vi "SM_DI-DAQInstrument.vi"(7 "DI TaskName":string, 8 "error in (no error)":errorcluster, 11 "DAQ Process AppData":T1) -> (0 "error out":errorcluster)   [LabVIEW 2017, in "DAQ.lvclass"]
doc: "Developed by Kevin Thompson\nkevin@thompsonengineering.net\n\nCopyright 2018-2020\nThompson Engineering, LLC"
uses:
  DAQ.lvclass
  Process_DAQ SM AppData--cluster.ctl
  DataTypes/TD DAQ Settings--cluster.ctl
  DataTypes/TD DI Instrument Settings--cluster.ctl
  DataTypes/TD AI Instrument Settings--cluster.ctl
  DataTypes/TD AI InstSettings--cluster.ctl
  TD SimAI Ranges--cluster.ctl
  <vilib>/TELLC/Dynamic CVT API/TD Dynamic CVT DVR--ref.ctl
  TD local raw DI Data--cluster.ctl
  <vilib>/DAQmx/read.llb/DAQmx Read (Digital 1D Bool NChan 1Samp 1Line).vi
  <vilib>/DAQmx/miscellaneous.llb/DAQmx Fill In Error Info.vi
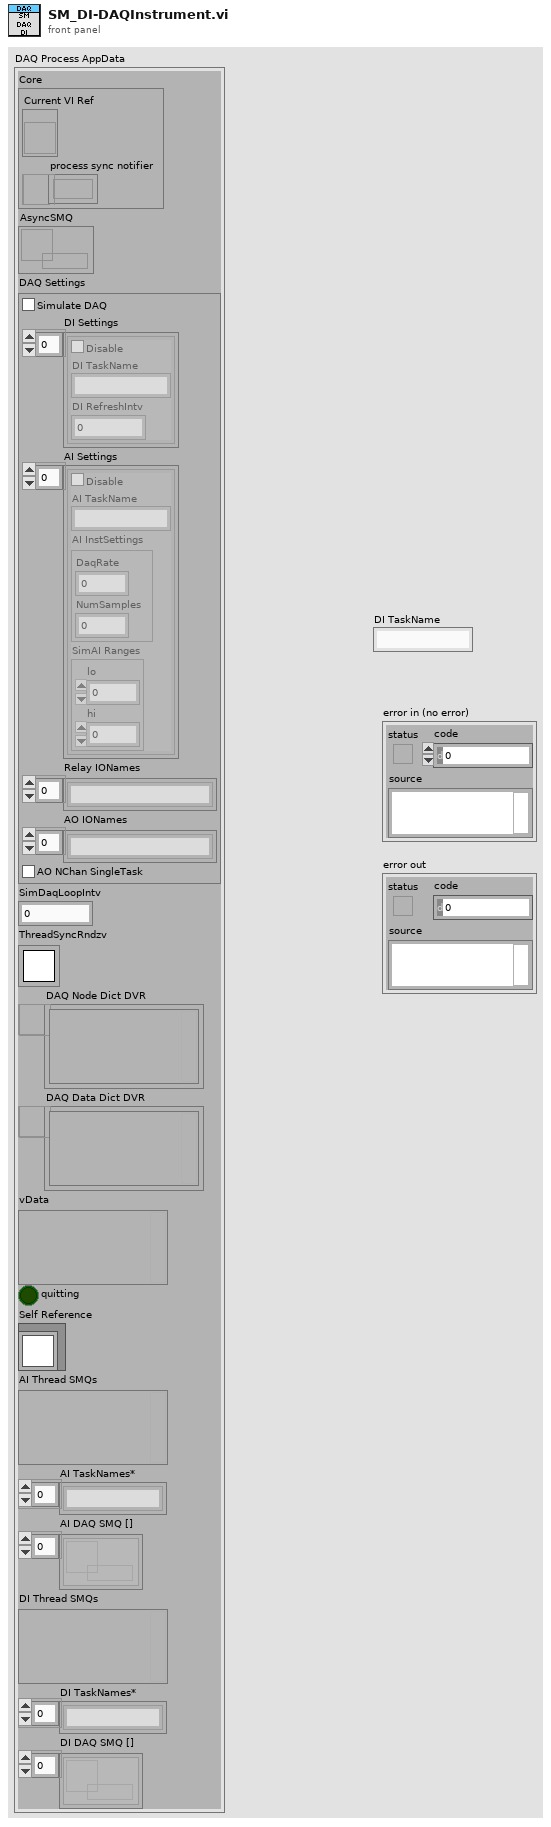
[diagram p1: front panel]
types:
  T1 = typedef "DAQ.lvclass/Process_DAQ SM AppData--cluster.ctl" = cluster{"Core":cluster{"Current VI Ref":refnum<vi>, "process sync notifier":refnum<notifier>}, "AsyncSMQ":refnum<queue>, "DAQ Settings":T2, "SimDaqLoopIntv":i32, "ThreadSyncRndzv":T7, "DAQ Node Dict DVR":T8, "DAQ Data Dict DVR":T8, "vData":variant, "quitting":bool, "Self Reference":refnum<class "DAQ.lvclass">, "AI Thread SMQs":variant, "AI TaskNames*":string[], "AI DAQ SMQ []":refnum<queue>[], "DI Thread SMQs":variant, "DI TaskNames*":string[], "DI DAQ SMQ []":refnum<queue>[]}
  T2 = typedef "DAQ.lvclass/TD DAQ Settings--cluster.ctl" = cluster{"Simulate DAQ":bool, "DI Settings":T3[], "AI Settings":T4[], "Relay IONames":string[], "AO IONames":string[], "AO NChan SingleTask":bool}
  T3 = typedef "DAQ.lvclass/TD DI Instrument Settings--cluster.ctl" = cluster{"Disable":bool, "DI TaskName":string, "DI RefreshIntv":i32}
  T4 = typedef "DAQ.lvclass/TD AI Instrument Settings--cluster.ctl" = cluster{"Disable":bool, "AI TaskName":string, "AI InstSettings":T5, "SimAI Ranges":T6}
  T5 = typedef "DAQ.lvclass/TD AI InstSettings--cluster.ctl" = cluster{"DaqRate":dbl, "NumSamples":i32}
  T6 = typedef "DAQ.lvclass/TD SimAI Ranges--cluster.ctl" = cluster{"lo":dbl, "hi":dbl}
  T7 = typedef "Rendezvous RefNum" = refnum<k1>
  T8 = typedef "TD Dynamic CVT DVR--ref.ctl" = refnum<data-value>
  T9 = cluster{"UpdateUIControl Ev":refnum<user-event>, "stop process Ev":refnum<user-event>, "change mode Ev":refnum<user-event>}
  T10 = typedef "DAQ.lvclass/TD DI local thread params--clustser.ctl" = cluster{"DI IONames":string[], "DAQ running":bool, "RawDIDataQ":refnum<queue>, "DI Local CmdQ":refnum<queue>, "DI TaskName":string, "DI Settings":T3, "NextTimerExp":dbl, "DI DAQTaskRef":refnum<k21>, "DI SMQ":refnum<queue>}
  T11 = cluster{"DAQ Process AppData":T1, "DI thread params":T10}
  T12 = typedef "DAQ.lvclass/TD local raw DI Data--cluster.ctl" = cluster{dbl, "data":bool[]}
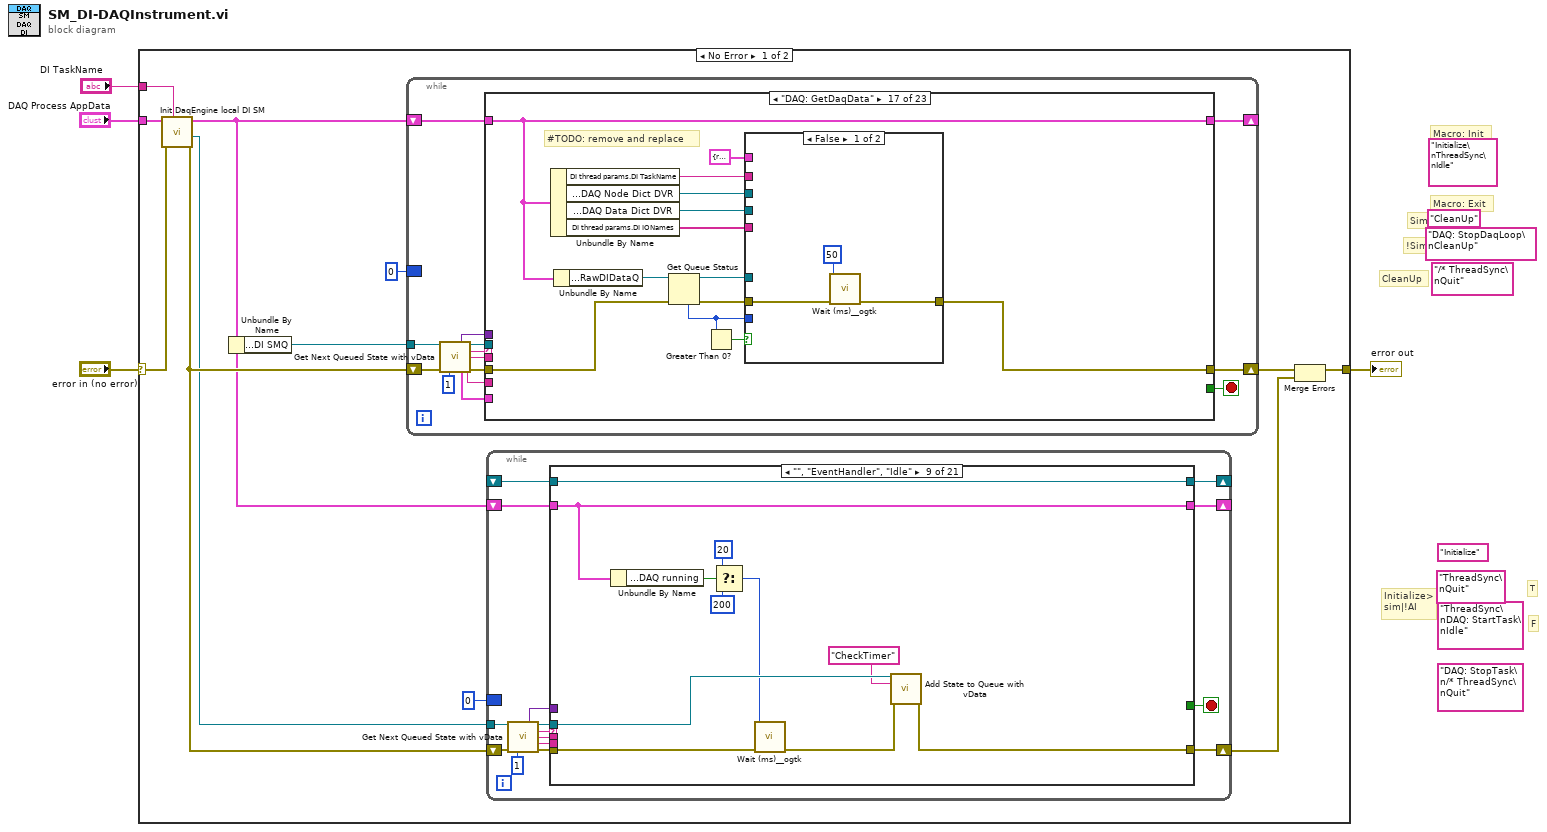
[diagram p0: block diagram]
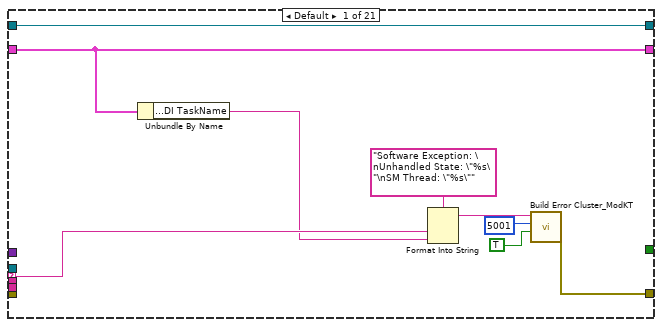
[diagram p2: hidden frame]
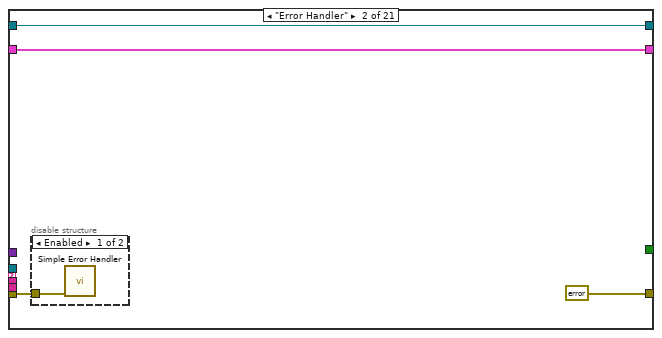
[diagram p3: hidden frame]
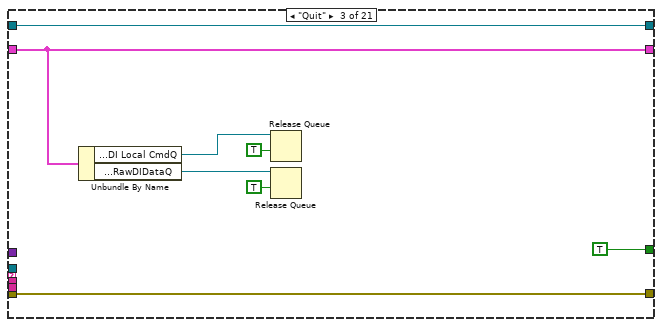
[diagram p5: hidden frame]
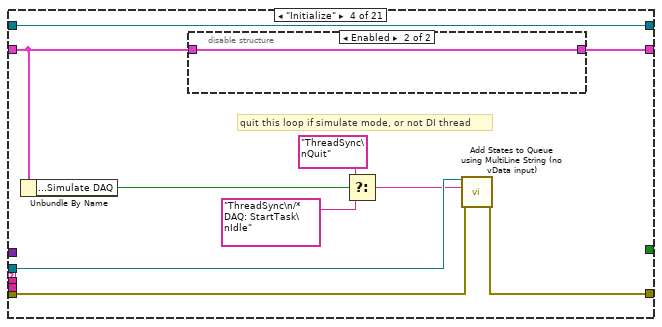
[diagram p6: hidden frame]
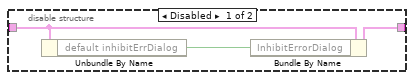
[diagram p7: hidden frame]
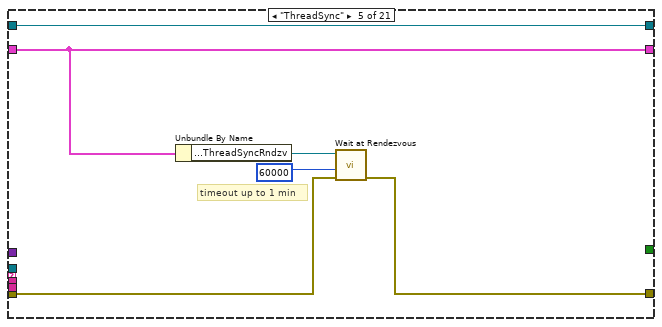
[diagram p8: hidden frame]
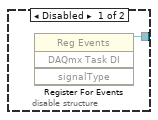
[diagram p10: hidden frame]
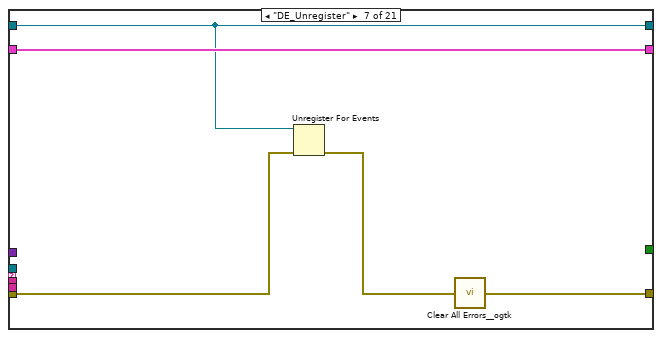
[diagram p11: hidden frame]
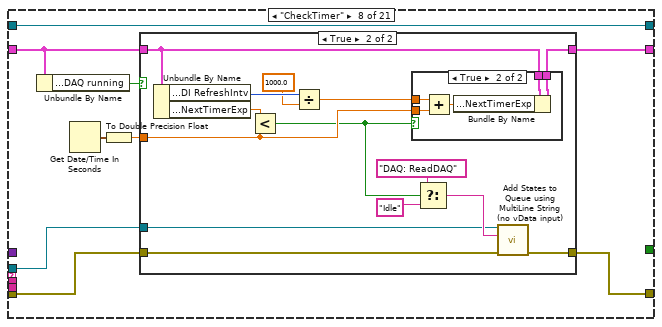
[diagram p12: hidden frame]
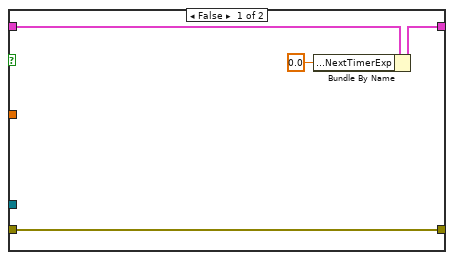
[diagram p13: hidden frame]
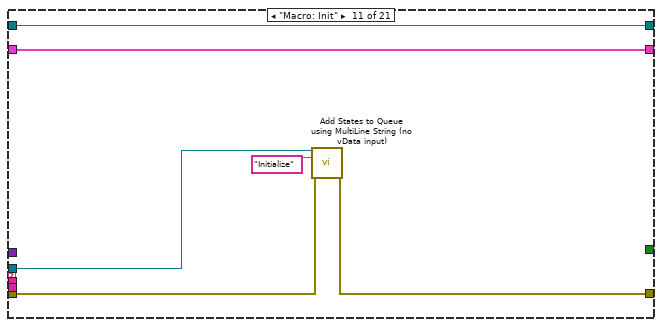
[diagram p16: hidden frame]
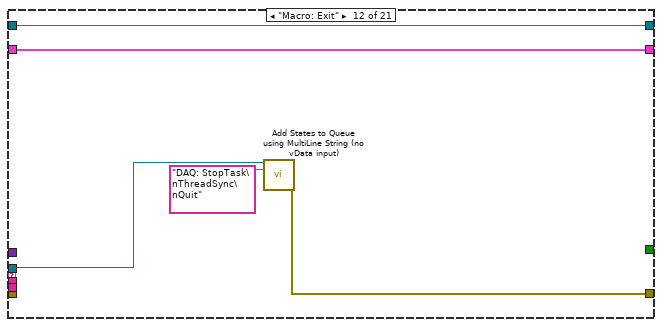
[diagram p17: hidden frame]
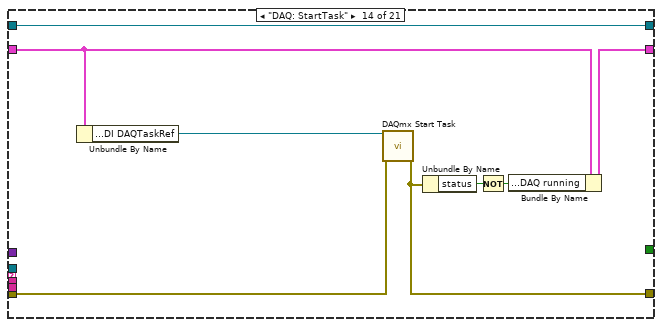
[diagram p19: hidden frame]
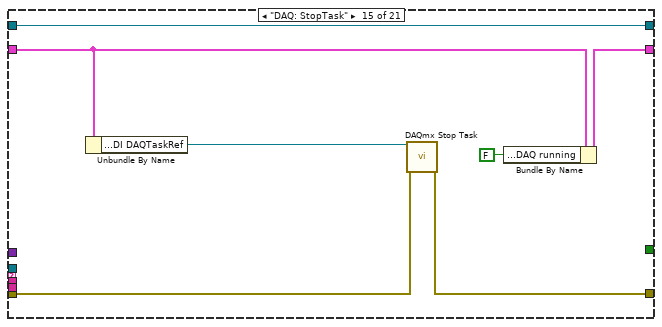
[diagram p20: hidden frame]
diagram:
  (unwired) "DAQ: StopTask\n/* ThreadSync\nQuit" ("states in")
  (unwired) "ThreadSync\nDAQ: StartTask\nIdle"
  (unwired) "Initialize" ("states in")
  (unwired) "ThreadSync\nQuit"
  (unwired) "/* ThreadSync\nQuit" ("states in")
  (unwired) "DAQ: StopDaqLoop\nCleanUp"
  (unwired) "CleanUp"
  (unwired) "Initialize\nThreadSync\nIdle"
  # "F"
  # "T"
  # "Initialize>\nsim|!AI"
  # "CleanUp"
  # "!Sim"
  # "Sim"
  # "Macro: Init"
  # "Macro: Exit"
  n1 = case shown="No Error" "error in (no error)" {
    selector: "error in (no error)" -> [w14 w455]
    tunnel: [w12 w455] -> w4
    tunnel: "DAQ Process AppData" -> [w15 _]
    tunnel: "DI TaskName" -> [w5 _]
    frame No Error {
      n2 = call "Init DaqEngine local DI SM.vi"("DI TaskName"=w5, "error in (no error)"=w14, "DAQ Process AppData"=w15) -> ("error out"=w13:errorcluster, "local LoopCmdQ"=w10:refnum<queue>, "DAQProcess DI AppData+"=w6:T11)  [unwired: 6 in]
      n3 = Unbundle By Name(w6) -> ("DI thread params.DI SMQ"=w7:refnum<queue>)
      n4 = while {
        shift-right: [w246] -> _
        shift-left: w6 -> [w255]
        shift-right: [w249] -> w16
        shift-left: w13 -> [w248]
        tunnel: w7 -> [w245]
        border: u32 0 ("millisecond timer value") -> [_]
        stop <- w251 stop-if-true
        n5 = call <vilib>:"Get Next Queued State with vData.vi"("queue in"=w245, "error in (no error)"=w248, "timeout (100)"=1) -> ("vData out"=w252:variant, "queue out"=w247:refnum<queue>, "Next State"=w254:string, "queued msg"=w253:string, "Prev State"=w243:string, "RemainingElements"=w244:cluster{"state":string, "vData":variant}[], "error out"=w250:errorcluster)  [unwired: 6 in]
        n6 = case shown="\"DAQ: GetDaqData\"" w254 {
          selector: w254 -> [w259 _ _ _ _ _ _ _ _ _ _ _ _ _ _ _ _ _ _ _ _ _ _]
          tunnel: w255 -> [w258 w266 w269 w272 w292 w299 w300 w305 w312 w316 w320 w325 w328 w335 w342 w345 w355 w397 w400 w407 w416 w421 w442]
          tunnel: w253 -> [_ _ _ _ _ _ _ _ _ _ _ _ _ _ _ _ _ _ _ w406 _ _ _]
          tunnel: w252 -> [_ _ _ _ _ _ _ _ _ _ _ _ _ _ _ _ _ _ _ _ w413 w422 w439]
          tunnel: w243 -> [_ _ _ _ _ _ _ _ _ _ _ _ _ _ _ _ _ _ _ _ _ _ _]
          tunnel: [FALSE _ TRUE _ _ _ _ _ _ _ _ _ _ _ _ _ _ _ _ _ _ _ _] -> w251
          tunnel: w250 -> [_ w265 w271 w274 w291 w296 _ w306 w311 w315 w318 w323 w331 w336 w341 w346 w356 w383 w399 w401 w418 w424 w441]
          tunnel: [w257 errorcluster {"status"=FALSE, "code"=0, "source"=""} ("error out") w271 w274 w290 w297 w301 w306 w313 w315 w317 w322 w329 w337 w341 w347 w350 w389 w399 w402 w411 w423 w440] -> w249
          tunnel: w247 -> [_ _ _ _ _ w295 _ _ w314 _ _ _ w330 w338 _ _ _ _ _ _ _ _ _]
          tunnel: [w258 w266 w269 w273 w292 w299 w300 w305 w312 w316 w320 w325 w328 w335 w342 w345 w355 w397 w400 w407 w410 w420 w438] -> w246
          tunnel: w244 -> [_ _ _ _ _ _ _ _ _ _ _ _ _ _ _ _ _ _ _ _ _ _ _]
          frame Default {
            n7 = Unbundle By Name(w258) -> ("DI thread params.DI TaskName"=w256:string)
            n8 = Format Into String(format string="Software Exception: \nUnhandled State: \"%s\"\nSM Thread: \"%s\"", w259, w256) -> (resulting string=w260:string)  [unwired: 2 in, 1 out]
            n9 = call <vilib>:"Build Error Cluster_ModKT .vi"("Prepend String (\"\")"=w260, "code"=5001, "error? (F)"=TRUE ("error?")) -> ("error out"=w257:errorcluster)  [unwired: 4 in, 1 out]
          }
          frame "Error Handler" {
            # "Note, this is an image"
            n10 = disable-structure shown="Enabled" {
              disable-tunnel: w265 -> [_ w268]
              frame Disabled {
              }
              frame Enabled {
                n11 = call <vilib>:"Simple Error Handler.vi"("error in (no error)"=w268) -> ()  [unwired: 4 in, 5 out]
              }
            }
          }
          frame "Quit" {
          }
          frame "Initialize" {
            n12 = disable-structure shown="Enabled" {
              disable-tunnel: [w277 w280 w289] -> w273
              disable-tunnel: w272 -> [w276 w281 w289]
              disable-tunnel: w272 -> [_ w284 _]
              frame Disabled {
                n13 = Unbundle By Name(w276) -> ("default inhibitErrDialog"=w275:bool)
                n14 = Bundle By Name(cluster=w276, "InhibitErrorDialog"=w275) -> (w277:T11)
              }
              frame Disabled {
                n15 = Unbundle By Name(w284) -> ("DI thread params.DI TaskName"=w278:string, "DAQ Process AppData.Self Reference"=w283:refnum<class "DAQ.lvclass">)
                n16 = property class="DAQ"(reference=w283) -> ("Accessors:DAQ Settings*"=w282:T2)  [unwired: 1 in, 2 out]
                n17 = Unbundle By Name(w282) -> ("DI Settings"=w279:T3[])
                n18 = for {
                  tunnel: w279 -> [w287] mode=indexing
                  tunnel: w278 -> [w286]
                  tunnel: [w287] -> _
                  stop <- w285 stop-if-true
                  n19 = Unbundle By Name(w287) -> ("DI TaskName"=w288:string)
                  n20 = Equal?(x=w286, y=w288) -> (x = y?=w285:bool)
                }
                n21 = Bundle By Name(cluster=w281) -> (w280:T11)  [unwired: 1 in]
              }
              frame Enabled {
              }
            }
          }
          frame "ThreadSync" {
            # "timeout up to 1 min"
            n22 = Unbundle By Name(w292) -> ("DAQ Process AppData.ThreadSyncRndzv"=w294:T7)
            n23 = call <vilib>:"Wait at Rendezvous.vi"("error in (no error)"=w291, "ms timeout (-1)"=60000, "rendezvous"=w294) -> ("error out"=w290:errorcluster)  [unwired: 2 in, 2 out]
          }
          frame "CleanUp" {
            n24 = call <vilib>:"Add States to Queue using MultiLine String (no vData input).vi"("queue in"=w295, "states in"="ThreadSync\nQuit", "error in"=w296) -> ("error out"=w297:errorcluster)  [unwired: 10 in, 2 out]
          }
          frame "SignalQuit" {
            n25 = disable-structure shown="Enabled" {
              disable-tunnel: [w303 errorcluster {"status"=FALSE, "code"=0, "source"=""} ("error constant")] -> w301
              disable-tunnel: w300 -> [w302 _]
              frame Disabled {
              }
              frame Enabled {
              }
            }
          }
          frame "CheckTimer" {
          }
          frame "", "Idle" {
            n26 = Unbundle By Name(w312) -> ("DAQ Process AppData.DAQ Settings.Simulate DAQ"=w310:bool)
            n27 = Select(t="DAQ: GetSimDaqData" ("state"), s=w310, f="DAQ: GetDaqData" ("state")) -> (s? t:f=w307:string)
            n28 = call <vilib>:"Add State to Queue with vData.vi"("queue in"=w314, "state in"=w307, "error in"=w311) -> ("error out"=w313:errorcluster)  [unwired: 9 in, 3 out]
          }
          frame "------ Macro ------" {
          }
          frame "Macro: StopDAQ" {
            n29 = Unbundle By Name(w320) -> ("DI thread params.DI Local CmdQ"=w319:refnum<queue>)
            n30 = call <vilib>:"Add States to Queue using MultiLine String (no vData input).vi"("queue in"=w319, "states in"="DAQ: StopTask\n/* DE_Unregister\nIdle", "error in"=w318) -> ("error out"=w317:errorcluster)  [unwired: 10 in, 2 out]
          }
          frame "Macro: StartDAQ" {
            n31 = Unbundle By Name(w325) -> ("DI thread params.DI Local CmdQ"=w324:refnum<queue>)
            n32 = call <vilib>:"Add States to Queue using MultiLine String (no vData input).vi"("queue in"=w324, "states in"="DAQ: StopTask\n/* DE_Unregister\n/* DAQ: ConfigDaq\nAction: Wait >> 200\n/* DE_Register\nDAQ: StartTask\nIdle", "error in"=w323) -> ("error out"=w322:errorcluster)  [unwired: 10 in, 2 out]
          }
          frame "Macro: Init" {
            n33 = call <vilib>:"Add States to Queue using MultiLine String (no vData input).vi"("queue in"=w330, "states in"="Initialize\nThreadSync\nIdle", "error in"=w331) -> ("error out"=w329:errorcluster)  [unwired: 10 in, 2 out]
          }
          frame "Macro: Exit" {
            n34 = Unbundle By Name(w335) -> ("DI thread params.DI Local CmdQ"=w334:refnum<queue>)
            n35 = Get Queue Status(queue=w334) -> (error out=w333:errorcluster)  [unwired: 2 in, 7 out]
            n36 = case shown="No Error" w333 {
              tunnel: ["DAQ: StopDaqLoop\nCleanUp" "CleanUp"] -> w332
              frame No Error {
              }
              frame Error {
              }
            }
            n37 = call <vilib>:"Add States to Queue using MultiLine String (no vData input).vi"("queue in"=w338, "states in"=w332, "error in"=w336) -> ("error out"=w337:errorcluster)  [unwired: 10 in, 2 out]
          }
          frame "------ DAQ ------" {
          }
          frame "DAQ: StopDaqLoop" {
            n38 = Unbundle By Name(w345) -> ("DI thread params.DI Local CmdQ"=w344:refnum<queue>)
            n39 = call <vilib>:"Add States to Queue using MultiLine String (no vData input).vi"("queue in"=w344, "states in"="Macro: Exit", "error in"=w346) -> ("error out"=w347:errorcluster)  [unwired: 10 in, 2 out]
          }
          frame "DAQ: GetDaqData" {
            # "#TODO: remove and replace"
            n40 = Unbundle By Name(w355) -> ("DI thread params.DI TaskName"=w351:string, "DAQ Process AppData.DAQ Node Dict DVR"=w352:T8, "DAQ Process AppData.DAQ Data Dict DVR"=w353:T8, "DI thread params.DI IONames"=w354:string[])
            n41 = Unbundle By Name(w355) -> ("DI thread params.RawDIDataQ"=w360:refnum<queue>)
            n42 = Get Queue Status(queue=w360, error in (no error)=w356) -> (queue out=w359:refnum<queue>, error out=w357:errorcluster, # elements in queue=w349:i32)  [unwired: 1 in, 5 out]
            n43 = Greater Than 0?(x=w349) -> (x > 0?=w358:bool)
            n44 = case shown="False" w358 {
              tunnel: w359 -> [_ w372]
              tunnel: w357 -> [w363 w371]
              tunnel: w354 -> [_ w367]
              tunnel: w353 -> [_ w368]
              tunnel: w352 -> [_ w369]
              tunnel: w351 -> [_ w370]
              tunnel: [w362 w366] -> w350
              tunnel: w349 -> [_ w365]
              tunnel: T9 {"UpdateUIControl Ev"=refnum, "stop process Ev"=refnum, "change mode Ev"=refnum} ("Public P&ID Events") -> [_ w364]
              frame False {
                n45 = call <userlib>:"Wait (ms)__ogtk.vi"("error in (no error)"=w363, "milliseconds to wait"=u32 50 ("wait (ms)")) -> ("error out"=w362:errorcluster)  [unwired: 8 in, 1 out]
              }
              frame True {
                n46 = for {
                  N: w365 -> [_]
                  tunnel: w372 -> [w380]
                  shift-right: [w378] -> w366
                  shift-left: w371 -> [w379]
                  tunnel: w370 -> [w377]
                  tunnel: w369 -> [w376]
                  tunnel: w368 -> [w375]
                  tunnel: w367 -> [w374]
                  tunnel: w364 -> [w373]
                  n47 = call "Read DI DAQ Data.vi"("DAQ Node Dict DVR"=w376, "DI TaskName"=w377, "Public P&ID Events"=w373, "DAQ Data Dict DVR"=w375, "DI IONames"=w374, "daqThread DI local Q"=w380, "error in"=w379) -> ("error out"=w378:errorcluster)  [unwired: 6 in, 2 out]
                }
              }
            }
          }
          frame "DAQ: GetSimDaqData" {
            # "compensate for state machine\nidle timeout (1 ms)"
            n48 = Unbundle By Name(w397) -> ("DI thread params.DI TaskName"=w390:string, "DAQ Process AppData.DAQ Node Dict DVR"=w396:T8, "DAQ Process AppData.DAQ Data Dict DVR"=w395:T8, "DI thread params.DI IONames"=w394:string[], "DI thread params.DI Settings.DI RefreshIntv"=w381:i32)
            n49 = Subtract(x=w381, y=u32 1) -> (x-y=w387:u32)
            n50 = In Range and Coerce(upper limit=u32 10000, x=w387, lower limit=u32 1) -> (coerced(x)=w386:u32)  [unwired: 1 out]
            n51 = call <userlib>:"Wait (ms)__ogtk.vi"("error in (no error)"=w383, "milliseconds to wait"=w386) -> ("error out"=w382:errorcluster)  [unwired: 8 in, 1 out]
            n52 = call "Sim Read DI DAQ Data.vi"("DaqDevice dCVT"=w396, "DI TaskName"=w390, "DaqData dCVT"=w395, "DI IONames"=w394, "error in"=w382) -> ("error out"=w389:errorcluster)  [unwired: 8 in, 2 out]
            n53 = stacked-sequence {
              tunnel: [w398] -> w393
              tunnel: w389 -> [_]
              frame #0 {
                n54 = Tick Count (ms)() -> (millisecond timer value=w398:u32)
              }
            }
            n55 = feedback #1() -> (w391:u32)
            n56 = feedback-in #1(w393) -> ()
            n57 = Subtract(x=w393, y=w391) -> (x-y=w392:u32)
            n58 = call "Update DaqLoopTimer Q.vi"("elapsed time (ms)"=w392, "AI TaskName"=w390) -> ()  [unwired: 6 in]
          }
          frame "------ Action ------" {
          }
          frame "Action: Wait" {
            n59 = Scan From String(format string="%d", input string=w406) -> (output 1=w404:i32)  [unwired: 3 in, 3 out]
            n60 = To Unsigned Long Integer(number=w404) -> (unsigned 32bit integer=w403:u32)
            n61 = call <userlib>:"Wait (ms)__ogtk.vi"("error in (no error)"=w401, "milliseconds to wait"=w403) -> ("error out"=w402:errorcluster)  [unwired: 8 in, 1 out]
          }
          frame "Action: UpdateInterval" {
            n62 = Variant To Data(error in=w418, type=u32 0, Variant=w413) -> (data=w414:u32, error out=w412:errorcluster)
            n63 = To Long Integer(number=w414) -> (32bit integer=w408:i32)
            n64 = Bundle By Name(cluster=w416, "DI thread params.DI Settings.DI RefreshIntv"=w408) -> (w410:T11)
            n65 = Unbundle By Name(w410) -> ("DI thread params.DI Local CmdQ"=w415:refnum<queue>)
            n66 = Unbundle By Name(w410) -> ("DAQ Process AppData.DAQ Settings.Simulate DAQ"=w409:bool)
            n67 = call <vilib>:"Add State to Queue with vData.vi"("queue in"=w415, "state in"="Action: UpdateInterval", "vData (\"\")"=w413, "bypass (F)"=w409, "error in"=w412) -> ("error out"=w411:errorcluster)  [unwired: 7 in, 3 out]
          }
          frame "Action: UpdateEnable" {
            n68 = disable-structure shown="Enabled" {
              disable-tunnel: w424 -> [w434 w436]
              disable-tunnel: [w430 w436] -> w423
              disable-tunnel: w422 -> [w429 _]
              disable-tunnel: w421 -> [w428 w437]
              disable-tunnel: [w426 w437] -> w420
              frame Disabled {
                n69 = Variant To Data(error in=w434, type=TRUE, Variant=w429) -> (data=w427:bool, error out=w431:errorcluster)
                n70 = Bundle By Name(cluster=w428, "DI"=w427) -> (w426:T11)
                n71 = Unbundle By Name(w426) -> ("DI thread params.DI Local CmdQ"=w432:refnum<queue>)
                n72 = Unbundle By Name(w426) -> ("DAQ Process AppData.DAQ Settings.Simulate DAQ"=w425:bool)
                n73 = call <vilib>:"Add State to Queue with vData.vi"("queue in"=w432, "state in"="Action: UpdateEnable", "vData (\"\")"=w429, "bypass (F)"=w425, "error in"=w431) -> ("error out"=w430:errorcluster)  [unwired: 7 in, 3 out]
              }
              frame Enabled {
              }
            }
          }
          frame "Action: SetInhibitErrDialog" {
            n74 = disable-structure shown="Enabled" {
              disable-tunnel: w442 -> [w453 _]
              disable-tunnel: w441 -> [w450 w454]
              disable-tunnel: [w446 w454] -> w440
              disable-tunnel: w439 -> [w445 _]
              disable-tunnel: [w444 _] -> w438
              frame Disabled {
                n75 = Variant To Data(error in=w450, type=FALSE, Variant=w445) -> (data=w451:bool, error out=w447:errorcluster)
                n76 = Bundle By Name(cluster=w453, "InhibitErrorDialog"=w451) -> (w444:T11)
                n77 = Unbundle By Name(w444) -> ("DAQ Process AppData.DAQ Settings.Simulate DAQ"=w443:bool)
                n78 = Unbundle By Name(w444) -> ("DI thread params.DI Local CmdQ"=w448:refnum<queue>)
                n79 = call <vilib>:"Add State to Queue with vData.vi"("queue in"=w448, "state in"="Action: SetInhibitErrDialog", "vData (\"\")"=w445, "bypass (F)"=w443, "error in"=w447) -> ("error out"=w446:errorcluster)  [unwired: 7 in, 3 out]
              }
              frame Enabled {
              }
            }
          }
        }
      }
      n80 = while {
        shift-right: [w27] -> _
        shift-left: _ -> [w26]
        shift-right: [w25] -> _
        shift-left: w6 -> [w31]
        shift-right: [w24] -> w11
        shift-left: w13 -> [w29]
        tunnel: w10 -> [w30]
        border: u32 0 ("millisecond timer value") -> [_]
        stop <- w18 stop-if-true
        n81 = call <vilib>:"Get Next Queued State with vData.vi"("queue in"=w30, "error in (no error)"=w29, "timeout (100)"=1) -> ("vData out"=w17:variant, "queue out"=w22:refnum<queue>, "Next State"=w21:string, "queued msg"=w20:string, "Prev State"=w19:string, "error out"=w28:errorcluster)  [unwired: 6 in, 1 out]
        n82 = case shown="\"\", \"EventHandler\", \"Idle\"" w21 {
          tunnel: w20 -> [_ _ _ _ _ _ _ _ _ _ _ _ _ _ _ _ _ w188 _ _ _]
          selector: w21 -> [w34 _ _ _ _ _ _ _ _ _ _ _ _ _ _ _ _ _ _ _ _]
          tunnel: w31 -> [w35 w43 w50 w57 w70 w77 w84 w90 w119 w130 w136 w141 w144 w152 w156 w166 w184 w192 w196 w202 w228]
          tunnel: w28 -> [_ w41 w52 w62 w69 w75 w82 w87 w127 w129 w134 _ w143 w146 w154 w168 w183 w187 w198 w206 w230]
          tunnel: [w40 w44 w53 w63 w73 w76 w83 w93 w128 w131 w137 w142 w145 w153 w160 w177 w185 w193 w201 w208 w232] -> w27
          tunnel: w26 -> [w40 w44 w53 w63 w73 w74 w83 w93 w128 w131 w137 w142 w145 w153 w160 w177 w185 w193 w201 w208 w232]
          tunnel: [w35 w43 w50 w56 w70 w77 w84 w89 w119 w130 w136 w141 w144 w151 w158 w166 w184 w192 w195 w205 w227] -> w25
          tunnel: [w33 errorcluster {"status"=FALSE, "code"=0, "source"=""} ("error out") w52 w61 w68 w75 w80 w88 w124 w129 w133 w139 w143 w150 w159 w173 w183 w186 w197 w204 w229] -> w24
          tunnel: w22 -> [_ _ _ w60 _ _ _ w86 w126 _ w132 w140 _ _ _ _ _ _ _ w203 _]
          tunnel: w19 -> [_ _ _ _ _ _ _ _ _ _ _ _ _ _ _ _ _ _ _ _ _]
          tunnel: [_ _ TRUE _ _ _ _ _ _ _ _ _ _ _ _ _ _ _ _ _ _] -> w18
          tunnel: w17 -> [_ _ _ _ _ _ _ _ _ _ _ _ _ _ _ _ _ _ w199 w207 w231]
          frame Default {
            n83 = Unbundle By Name(w35) -> ("DI thread params.DI TaskName"=w32:string)
            n84 = Format Into String(format string="Software Exception: \nUnhandled State: \"%s\"\nSM Thread: \"%s\"", w34, w32) -> (resulting string=w39:string)  [unwired: 2 in, 1 out]
            n85 = call <vilib>:"Build Error Cluster_ModKT .vi"("Prepend String (\"\")"=w39, "code"=5001, "error? (F)"=TRUE ("error?")) -> ("error out"=w33:errorcluster)  [unwired: 4 in, 1 out]
          }
          frame "Error Handler" {
            n86 = disable-structure shown="Enabled" {
              disable-tunnel: w41 -> [w45 _]
              frame Enabled {
                n87 = call <vilib>:"Simple Error Handler.vi"("error in (no error)"=w45) -> ()  [unwired: 4 in, 5 out]
              }
              frame Disabled {
              }
            }
          }
          frame "Quit" {
            n88 = Unbundle By Name(w50) -> ("DI thread params.DI Local CmdQ"=w46:refnum<queue>, "DI thread params.RawDIDataQ"=w48:refnum<queue>)
            n89 = Release Queue(queue=w46, force destroy? (F)=TRUE) -> ()  [unwired: 1 in, 3 out]
            n90 = Release Queue(queue=w48, force destroy? (F)=TRUE) -> ()  [unwired: 1 in, 3 out]
          }
          frame "Initialize" {
            # "quit this loop if simulate mode, or not DI thread"
            n91 = Unbundle By Name(w57) -> ("DAQ Process AppData.DAQ Settings.Simulate DAQ"=w55:bool)
            n92 = disable-structure shown="Enabled" {
              disable-tunnel: w57 -> [w66 w67]
              disable-tunnel: [w65 w67] -> w56
              frame Disabled {
                n93 = Unbundle By Name(w66) -> ("default inhibitErrDialog"=w64:bool)
                n94 = Bundle By Name(cluster=w66, "InhibitErrorDialog"=w64) -> (w65:T11)
              }
              frame Enabled {
              }
            }
            n95 = Select(t="ThreadSync\nQuit", s=w55, f="ThreadSync\n/* DAQ: StartTask\nIdle") -> (s? t:f=w59:string)
            n96 = call <vilib>:"Add States to Queue using MultiLine String (no vData input).vi"("queue in"=w60, "states in"=w59, "error in"=w62) -> ("error out"=w61:errorcluster)  [unwired: 10 in, 2 out]
          }
          frame "ThreadSync" {
            # "timeout up to 1 min"
            n97 = Unbundle By Name(w70) -> ("DAQ Process AppData.ThreadSyncRndzv"=w71:T7)
            n98 = call <vilib>:"Wait at Rendezvous.vi"("error in (no error)"=w69, "ms timeout (-1)"=60000, "rendezvous"=w71) -> ("error out"=w68:errorcluster)  [unwired: 2 in, 2 out]
          }
          frame "DE_Register" {
            n99 = disable-structure shown="Enabled" {
              disable-tunnel: w77 -> [_ _]
              disable-tunnel: [w78 w79] -> w76
              disable-tunnel: w74 -> [_ w79]
              frame Disabled {
                n100 = register-events() -> (reference out=w78:refnum<event-registration>)  [unwired: 4 in, 1 out]
              }
              frame Enabled {
              }
            }
          }
          frame "DE_Unregister" {
            n101 = Unregister For Events(event registration refnum=w83, error in=w82) -> (error out=w81:errorcluster)
            n102 = call <userlib>:"Clear All Errors__ogtk.vi"("Error In"=w81) -> ("Error Out"=w80:errorcluster)  [unwired: 3 in]
          }
          frame "CheckTimer" {
            n103 = Unbundle By Name(w90) -> ("DI thread params.DAQ running"=w85:bool)
            n104 = Get Date/Time In Seconds() -> (seconds since 1Jan1904=w92:timestamp)
            n105 = To Double Precision Float(number=w92) -> (double precision float=w91:dbl)
            n106 = case shown="True" w85 {
              tunnel: w91 -> [_ w108]
              tunnel: w90 -> [w96 w98]
              tunnel: [w95 w106] -> w89
              tunnel: w86 -> [_ w101]
              tunnel: w87 -> [w97 w100]
              tunnel: [w97 w99] -> w88
              frame False {
                n107 = Bundle By Name(cluster=w96, "DI thread params.NextTimerExp"=0.0) -> (w95:T11)
              }
              frame True {
                n108 = Unbundle By Name(w98) -> ("DI thread params.DI Settings.DI RefreshIntv"=w111:i32, "DI thread params.NextTimerExp"=w107:dbl)
                n109 = Less?(x=w107, y=w108) -> (x < y?=w105:bool)
                n110 = Divide(x=w111, y=1000.0) -> (x/y=w109:dbl)
                n111 = case shown="True" w105 {
                  tunnel: w109 -> [_ w116]
                  tunnel: w98 -> [w112 w117]
                  tunnel: w108 -> [_ w114]
                  tunnel: [w112 w113] -> w106
                  frame False {
                  }
                  frame True {
                    n112 = Add(x=w116, y=w114) -> (x+y=w115:dbl)
                    n113 = Bundle By Name(cluster=w117, "DI thread params.NextTimerExp"=w115) -> (w113:T11)
                  }
                }
                n114 = Select(t="DAQ: ReadDAQ", s=w105, f="Idle") -> (s? t:f=w102:string)
                n115 = call <vilib>:"Add States to Queue using MultiLine String (no vData input).vi"("queue in"=w101, "states in"=w102, "error in"=w100) -> ("error out"=w99:errorcluster)  [unwired: 10 in, 2 out]
              }
            }
          }
          frame "", "EventHandler", "Idle" {
            n116 = Unbundle By Name(w119) -> ("DI thread params.DAQ running"=w118:bool)
            n117 = Select(t=u32 20 ("wait (ms)"), s=w118, f=u32 200) -> (s? t:f=w122:u32)
            n118 = call <userlib>:"Wait (ms)__ogtk.vi"("error in (no error)"=w127, "milliseconds to wait"=w122) -> ("error out"=w125:errorcluster)  [unwired: 8 in, 1 out]
            n119 = call <vilib>:"Add State to Queue with vData.vi"("queue in"=w126, "state in"="CheckTimer", "error in"=w125) -> ("error out"=w124:errorcluster)  [unwired: 9 in, 3 out]
          }
          frame "------ Macro ------" {
          }
          frame "Macro: Init" {
            n120 = call <vilib>:"Add States to Queue using MultiLine String (no vData input).vi"("queue in"=w132, "states in"="Initialize", "error in"=w134) -> ("error out"=w133:errorcluster)  [unwired: 10 in, 2 out]
          }
          frame "Macro: Exit" {
            n121 = call <vilib>:"Add States to Queue using MultiLine String (no vData input).vi"("queue in"=w140, "states in"="DAQ: StopTask\nThreadSync\nQuit") -> ("error out"=w139:errorcluster)  [unwired: 11 in, 2 out]
          }
          frame "------ DAQ ------" {
          }
          frame "DAQ: StartTask" {
            n122 = Unbundle By Name(w152) -> ("DI thread params.DI DAQTaskRef"=w147:refnum<k21>)
            n123 = call <vilib>:"DAQmx Start Task.vi"("task/channels in"=w147, "error in"=w146) -> ("error out"=w150:errorcluster)  [unwired: 12 in, 1 out]
            n124 = Unbundle By Name(w150) -> ("status"=w149:bool)
            n125 = Not(x=w149) -> (.not. x?=w148:bool)
            n126 = Bundle By Name(cluster=w152, "DI thread params.DAQ running"=w148) -> (w151:T11)
          }
          frame "DAQ: StopTask" {
            n127 = Unbundle By Name(w156) -> ("DI thread params.DI DAQTaskRef"=w155:refnum<k21>)
            n128 = call <vilib>:"DAQmx Stop Task.vi"("task/channels in"=w155, "error in"=w154) -> ("error out"=w159:errorcluster)  [unwired: 12 in, 1 out]
            n129 = Bundle By Name(cluster=w156, "DI thread params.DAQ running"=FALSE) -> (w158:T11)
          }
          frame "DAQ: ReadDAQ" {
            w164 = T12 {0.0, "data"=[]}  # Raw DI Data
            n130 = stacked-sequence {
              tunnel: [w179] -> w169
              tunnel: w168 -> [w178]
              tunnel: [w178] -> w162
              frame #0 {
                n131 = Tick Count (ms)() -> (millisecond timer value=w179:u32)
              }
            }
            n132 = Unbundle By Name(w166) -> ("DI thread params.RawDIDataQ"=w165:refnum<queue>, "DI thread params.DI DAQTaskRef"=w161:refnum<k21>, "DI thread params.DI TaskName"=w163:string)
            n133 = feedback #2() -> (w170:u32)
            n134 = feedback-in #2(w169) -> ()
            n135 = Subtract(x=w169, y=w170) -> (x-y=w167:u32)
            n136 = call "Update DaqLoopTimer Q.vi"("elapsed time (ms)"=w167, "AI TaskName"=w163) -> ()  [unwired: 6 in]
            n137 = call-poly <vilib>:"DAQmx Read.vi"("task/channels in"=w161, "error in"=w162) -> ("data"=w172:bool[], "error out"=w174:errorcluster)  [unwired: 11 in, 1 out]
            n138 = stacked-sequence {
              tunnel: [w181] -> w176
              tunnel: w172 -> [w180]
              tunnel: [w180] -> w171
              frame #0 {
                n139 = Get Date/Time In Seconds() -> (seconds since 1Jan1904=w182:timestamp)
                n140 = To Double Precision Float(number=w182) -> (double precision float=w181:dbl)
              }
            }
            n141 = Bundle(cluster=w164, w176, "data"=w171) -> (w175:T12)
            n142 = Enqueue Element(queue=w165, element=w175, error in (no error)=w174) -> (error out=w173:errorcluster)  [unwired: 1 in, 2 out]
          }
          frame "------ Action ------" {
          }
          frame "Action: Wait" {
            n143 = Scan From String(format string="%d", input string=w188) -> (output 1=w190:i32)  [unwired: 3 in, 3 out]
            n144 = To Unsigned Long Integer(number=w190) -> (unsigned 32bit integer=w189:u32)
            n145 = call <userlib>:"Wait (ms)__ogtk.vi"("error in (no error)"=w187, "milliseconds to wait"=w189) -> ("error out"=w186:errorcluster)  [unwired: 8 in, 1 out]
          }
          frame "Action: UpdateInterval" {
            n146 = Variant To Data(error in=w198, type=u32 0, Variant=w199) -> (data=w194:u32, error out=w197:errorcluster)
            n147 = Bundle By Name(cluster=w196, "DI thread params.DI Settings.DI RefreshIntv"=w194) -> (w195:T11)
          }
          frame "Action: UpdateEnable" {
            n148 = disable-structure shown="Disabled" {
              disable-tunnel: w207 -> [w222 _]
              disable-tunnel: w206 -> [w221 w226]
              disable-tunnel: [w220 _] -> w205
              disable-tunnel: [w215 w226] -> w204
              disable-tunnel: w203 -> [w214 _]
              disable-tunnel: w202 -> [w213 _]
              frame Disabled {
                n149 = Unbundle By Name(w213) -> ("DI"=w209:bool)
                n150 = Variant To Data(error in=w221, type=TRUE, Variant=w222) -> (data=w211:bool, error out=w216:errorcluster)
                n151 = Not Exclusive Or(1:w211, 2:w209) -> (0:w212:bool)
                n152 = Select(t="DAQ: StartTask", s=w211, f="DAQ: StopTask") -> (s? t:f=w217:string)
                n153 = stacked-sequence {
                  tunnel: w213 -> [w225]
                  tunnel: [w224] -> w220
                  tunnel: w211 -> [w223]
                  frame #0 {
                    n154 = Bundle By Name(cluster=w225, "DI"=w223) -> (w224:T11)
                  }
                }
                n155 = call <vilib>:"Add State to Queue with vData.vi"("queue in"=w214, "state in"=w217, "bypass (F)"=w212, "error in"=w216) -> ("error out"=w215:errorcluster)  [unwired: 8 in, 3 out]
              }
              frame Enabled {
              }
            }
          }
          frame "Action: SetInhibitErrDialog" {
            n156 = disable-structure shown="Enabled" {
              disable-tunnel: w231 -> [w238 _]
              disable-tunnel: w230 -> [w237 w241]
              disable-tunnel: [w236 w241] -> w229
              disable-tunnel: w228 -> [w235 w240]
              disable-tunnel: [w234 w240] -> w227
              frame Disabled {
                n157 = Variant To Data(error in=w237, type=TRUE, Variant=w238) -> (data=w233:bool, error out=w236:errorcluster)
                n158 = Bundle By Name(cluster=w235, "InhibitErrorDialog"=w233) -> (w234:T11)
              }
              frame Enabled {
              }
            }
          }
        }
      }
      n159 = Merge Errors(w16, w11) -> (w12:errorcluster)
    }
    frame Error {
    }
  }
  "error out" <- w4
